vi "Zero setting for galvo module.vi"() -> ()   [LabVIEW 2025]
uses:
  <vilib>/DAQmx/write.llb/DAQmx Write (Analog 1D DBL NChan 1Samp).vi
  <vilib>/DAQmx/create/channels.llb/DAQmx Create Channel (AO-Voltage-Basic).vi
  <vilib>/DAQmx/miscellaneous.llb/DAQmx Fill In Error Info.vi
panel:
  in  "String":string
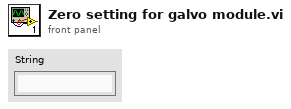
[diagram p1: front panel]
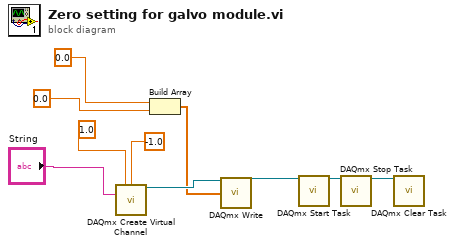
[diagram p0: block diagram]
diagram:
  n1 = call-poly <vilib>:"DAQmx Create Virtual Channel.vi"("maximum value"=1.0 ("minimum value"), "minimum value"=-1.0, "physical channels"="String") -> ("task out"=w7:refnum<k21>)  [unwired: 11 in, 1 out]
  n2 = Build Array(0.0 ("element"), 0.0 ("element")) -> (w3:dbl[])
  n3 = call-poly <vilib>:"DAQmx Write.vi"("task/channels in"=w7, "data"=w3) -> ("task out"=w8:refnum<k21>)  [unwired: 11 in, 2 out]
  n4 = call <vilib>:"DAQmx Start Task.vi"("task/channels in"=w8) -> ("task out"=w9:refnum<k21>)  [unwired: 13 in, 1 out]
  n5 = call <vilib>:"DAQmx Stop Task.vi"("task/channels in"=w9) -> ("task out"=w10:refnum<k21>)  [unwired: 13 in, 1 out]
  n6 = call <vilib>:"DAQmx Clear Task.vi"("task in"=w10) -> ()  [unwired: 14 in, 1 out]
